vi "prim_lt.vi"(11 "arguments":T1[](array[typedef])) -> (3 "Expression out":T1)   [LabVIEW 2021]
uses:
  Expression.ctl
  ExpressionType.ctl
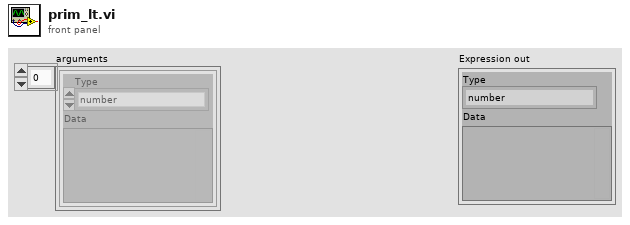
[diagram p1: front panel]
types:
  T1 = typedef "Expression.ctl" = cluster{"Type":T2, "Data":variant}
  T2 = typedef "ExpressionType.ctl" = enum16{"number", "string", "symbol", "primitive", "list", "closure", "macro", "nil", "error"}
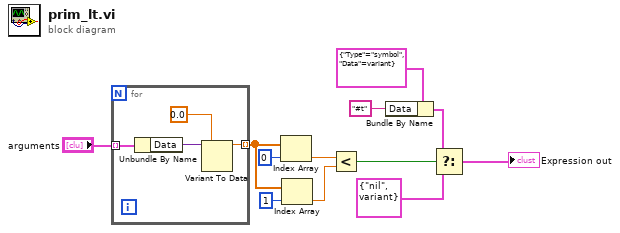
[diagram p0: block diagram]
diagram:
  n1 = for {
    tunnel: "arguments" -> [w16] mode=indexing
    tunnel: [w13] -> w9 mode=indexing
    n2 = Unbundle By Name(w16) -> ("Data"=w15:variant)
    n3 = Variant To Data(type=0.0, Variant=w15) -> (data=w13:dbl)  [unwired: 1 in, 1 out]
  }
  n4 = Index Array(array=w9, index=0) -> (element=w8:dbl)
  n5 = Index Array(array=w9, index=1) -> (element=w7:dbl)
  n6 = Less?(x=w8, y=w7) -> (x < y?=w6:bool)
  n7 = Bundle By Name(cluster=T1 {"Type"=enum."symbol", "Data"=variant} ("Expression 3"), "Data"="#t") -> (w3:T1)
  n8 = Select(t=w3, s=w6, f=T1 {"Type"=enum."nil", "Data"=variant} ("Expression 3")) -> (s? t:f=→"Expression out":T1)
